vi "CalcMagnitude2.vi"(8 "input valid":bool=TRUE, 11 "Data in":fxp<+/-,32,14>[](array[numeric])=[0.0, 0.0]) -> (0 "output valid":bool, 2 "Amp1":fxp<+,16,14>)   [LabVIEW 2018]
uses:
  <vilib>/rvi/FXPMathLib/FxpSqrt/subVIs/nifxpmath_Sqrt_SimConfig.ctl
  <vilib>/fxp/LVFixedPointOverflowPolicyTypeDef.ctl
  <vilib>/rvi/FXPMathLib/FxpSqrt/simVIs/DllSqrtTemp_sub.vi
  <vilib>/rvi/FXPMathLib/FxpAdd/XNode/nifxpmath_Add.xnode
  <vilib>/rvi/FXPMathLib/FxpSqrt/XNode/nifxpmath_Sqrt.xnode
  <vilib>/rvi/FXPMathLib/FxpMul/XNode/nifxpmath_Multiplier.xnode
  <vilib>/rvi/FXPMathLib/sim/FxpSim.dll
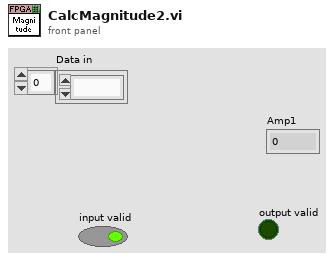
[diagram p1: front panel]
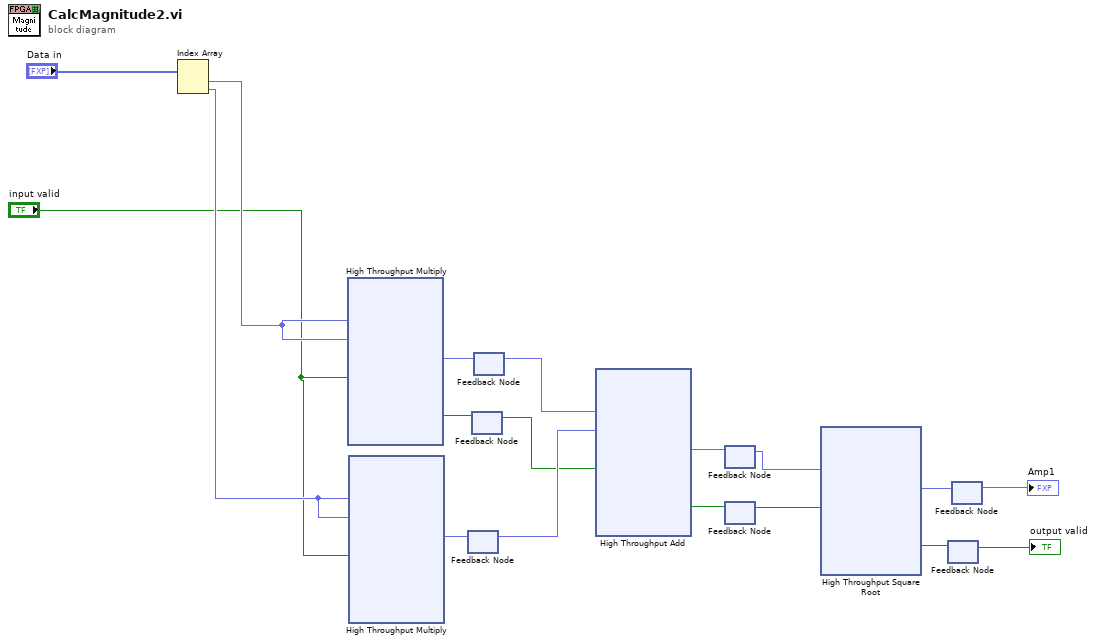
[diagram p0: block diagram]
diagram:
  n1 = Index Array(array="Data in") -> (element #1=w6:fxp<+/-,32,14>, element #2=w5:fxp<+/-,32,14>)  [unwired: 2 in]
  n2 = xnode "High Throughput Multiply"("x"=w6, "y"=w6, "input valid"="input valid") -> ("x*y"=w9:fxp<+,32,28>, "output valid"=w7:bool)  [unwired: 1 in, 1 out]
  n3 = xnode "High Throughput Multiply"("x"=w5, "y"=w5, "input valid"="input valid") -> ("x*y"=w11:fxp<+,32,28>)  [unwired: 1 in, 2 out]
  n4 = feedback #1() -> (w12:fxp<+,32,28>)  [unwired: 1 in]
  n5 = feedback-in #1(w11) -> ()
  n6 = feedback #2() -> (w8:bool)  [unwired: 1 in]
  n7 = feedback-in #2(w7) -> ()
  n8 = feedback #3() -> (w10:fxp<+,32,28>)  [unwired: 1 in]
  n9 = feedback-in #3(w9) -> ()
  n10 = xnode "High Throughput Add"("x"=w10, "y"=w12, "input valid"=w8) -> ("x+y"=w15:fxp<+,32,28>, "output valid"=w13:bool)  [unwired: 1 in, 1 out]
  n11 = feedback #4() -> (w16:fxp<+,32,28>)  [unwired: 1 in]
  n12 = feedback-in #4(w15) -> ()
  n13 = feedback #5() -> (w14:bool)  [unwired: 1 in]
  n14 = feedback-in #5(w13) -> ()
  n15 = xnode "High Throughput Square Root"("x"=w16, "input valid"=w14) -> ("sqrt(x)"=w17:fxp<+,16,14>, "output valid"=w2:bool)  [unwired: 1 in, 1 out]
  n16 = feedback #6() -> (→"output valid":bool)  [unwired: 1 in]
  n17 = feedback-in #6(w2) -> ()
  n18 = feedback #7() -> (→"Amp1":fxp<+,16,14>)  [unwired: 1 in]
  n19 = feedback-in #7(w17) -> ()
